vi "Add UID To Parent List.vi"(0 "Base Tree in":refnum<class "Base Tree.lvclass">, 1 "UID":string, 2 "Parent":string, 3 "error in (no error)":errorcluster) -> (7 "Base Tree out":refnum<class "Base Tree.lvclass">, 10 "error out":errorcluster)   [LabVIEW 2017, in "Browser Core.lvlib" / "Base Tree.lvclass"]
doc: "Add UID to the list of Children of the Parent Class"
uses:
  Base Tree.lvclass
  Base Tree.lvclass/Base Tree.ctl
  Node Classes/Generic Node/Generic Node.lvclass
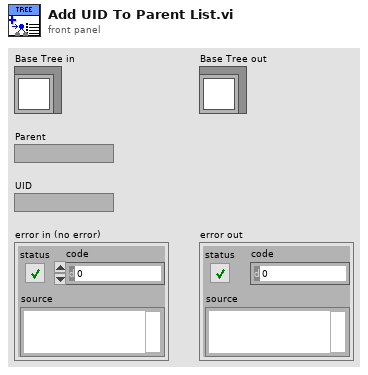
[diagram p1: front panel]
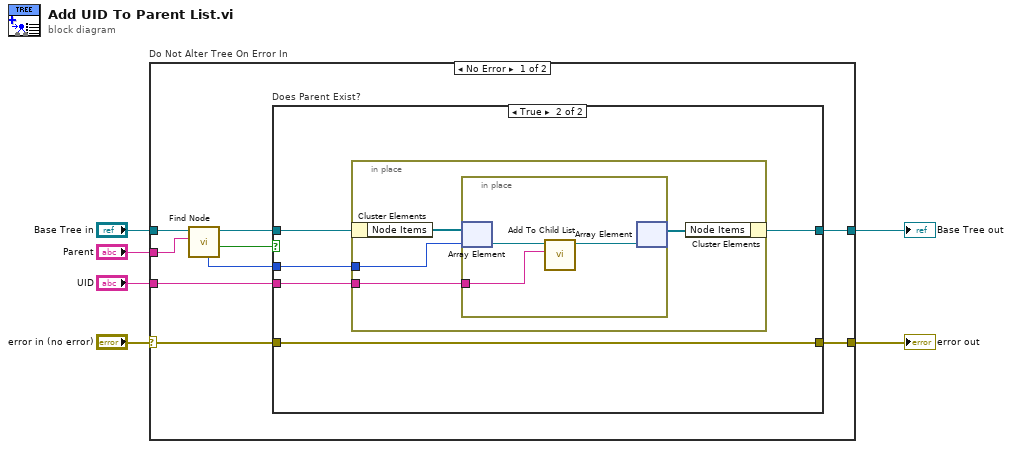
[diagram p0: block diagram]
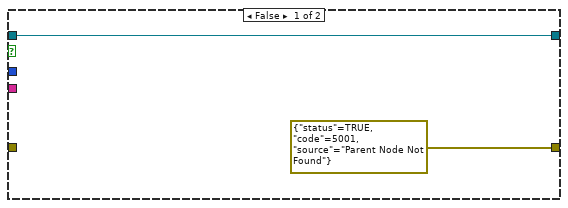
[diagram p2: hidden frame]
diagram:
  n1 = case "Do Not Alter Tree On Error In" shown="No Error" "error in (no error)" {
    selector: "error in (no error)" -> [w11 w30]
    tunnel: "Parent" -> [w15 _]
    tunnel: [w14 w31] -> w5
    tunnel: "Base Tree in" -> [w13 w31]
    tunnel: [w10 w30] -> w2
    tunnel: "UID" -> [w7 _]
    frame No Error {
      n2 = call-dynamic "Find Node.vi"("UID"=w15, "Base Tree in"=w13) -> ("Found?"=w9:bool, "Base Tree out"=w12:refnum<class "Base Tree.lvclass">, "Node Index"=w8:i32)  [unwired: 5 in, 2 out]
      n3 = case "Does Parent Exist?" shown="True" w9 {
        tunnel: [w16 w21] -> w14
        tunnel: w12 -> [w16 w22]
        tunnel: w11 -> [_ w18]
        tunnel: [errorcluster {"status"=TRUE, "code"=5001, "source"="Parent Node Not Found"} ("error in (no error)") w18] -> w10
        tunnel: w8 -> [_ w20]
        tunnel: w7 -> [_ w19]
        frame False {
        }
        frame True {
          n4 = in-place {
            in-place-border: w20 -> [w25]
            in-place-border: w19 -> [w23]
            n5 = in-place-cluster #1(w22) -> ("Node Items"=w26:refnum<class "Generic Node.lvclass">[])
            n6 = in-place {
              in-place-border: w23 -> [w28]
              n7 = in-place-array #2(w26, w25) -> (w29:refnum<class "Generic Node.lvclass">)
              n8 = call-dynamic "Add To Child List.vi"("Child ID"=w28, "Generic Node in"=w29) -> ("Generic Node out"=w27:refnum<class "Generic Node.lvclass">)  [unwired: 9 in]
              n9 = in-place-array #2(w27) -> (w24:refnum<class "Generic Node.lvclass">[])  [unwired: 1 out]
            }
            n10 = in-place-cluster #1("Node Items"=w24) -> (w21:refnum<class "Base Tree.lvclass">)
          }
        }
      }
    }
    frame Error {
    }
  }
  "Base Tree out" <- w5
  "error out" <- w2
